vi "PichAngle.vi"() -> ()   [LabVIEW 2016]
uses:
  Globals/Globals.vi
panel:
  out "Boolean":bool
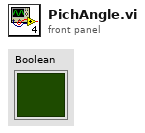
[diagram p1: front panel]
types:
  T1 = typedef "WPI_DigitalOutputDevRef.ctl" = cluster{"DIO Channel":T2, "DevStatus":errorcluster}
  T2 = typedef "FPGA_DIOChannel.ctl" = enum8{"DIO 0", "DIO 1", "DIO 2", "DIO 3", "DIO 4", "DIO 5", "DIO 6", "DIO 7", "DIO 8", "DIO 9", "DIO MXP 0", "DIO MXP 1", "DIO MXP 2", "DIO MXP 3", "DIO MXP 4", "DIO MXP 5", "DIO MXP 6", "DIO MXP 7", "DIO MXP 8", "DIO MXP 9", "DIO MXP 10", "DIO MXP 11", "DIO MXP 12", "DIO MXP 13", "DIO MXP 14", "DIO MXP 15", "SPI Port CS1", "SPI Port CS2", "SPI Port CS3", "SPI Port MISO", "SPI Port MOSI", "Invalid"}
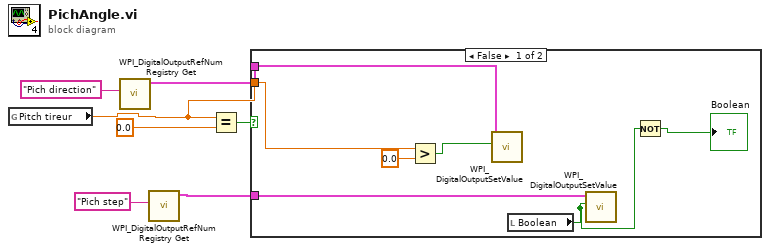
[diagram p0: block diagram]
diagram:
  n1 = global read "Globals.vi" "Pitch tireur"() -> (w3:dbl)
  n2 = call <vilib>:"WPI_DigitalOutputRefNum Registry Get.vi"("refnum name"="Pich direction") -> ("DigitalOutputDevRef"=w2:T1)  [unwired: 9 in, 1 out]
  n3 = call <vilib>:"WPI_DigitalOutputRefNum Registry Get.vi"("refnum name"="Pich step") -> ("DigitalOutputDevRef"=w1:T1)  [unwired: 9 in, 1 out]
  n4 = Equal?(x=w3, y=0.0) -> (x = y?=w4:bool)
  n5 = case shown="False" w4 {
    tunnel: w3 -> [w14 _]
    tunnel: w2 -> [w11 _]
    tunnel: w1 -> [w10 _]
    frame False {
      n6 = Greater?(x=w14, y=0.0) -> (0:w12:bool)
      n7 = call <vilib>:"WPI_DigitalOutputSetValue.vi"("Value"=w12, "DigitalOutputDevRef"=w11) -> ()  [unwired: 8 in, 2 out]
      n8 = local read "Boolean"() -> (w9:bool)
      n9 = call <vilib>:"WPI_DigitalOutputSetValue.vi"("Value"=w9, "DigitalOutputDevRef"=w10) -> ()  [unwired: 8 in, 2 out]
      n10 = Not(x=w9) -> (.not. x?=→"Boolean":bool)
    }
    frame True {
    }
  }
